vi "小灯泡控制pro.vi"() -> ()   [LabVIEW 2019]
panel:
  out "数值":i32
  out "布尔 2":bool
  in  "布尔":bool
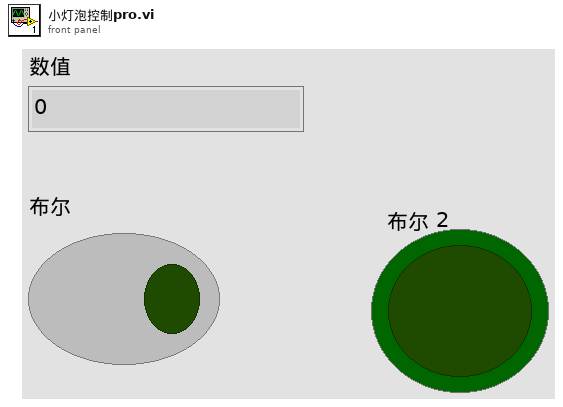
[diagram p1: front panel]
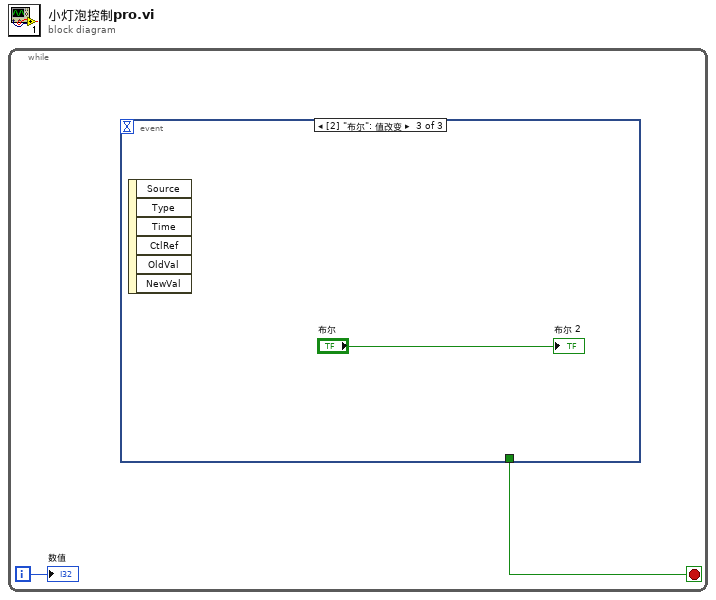
[diagram p0: block diagram]
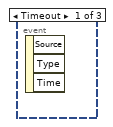
[diagram p2: hidden frame]
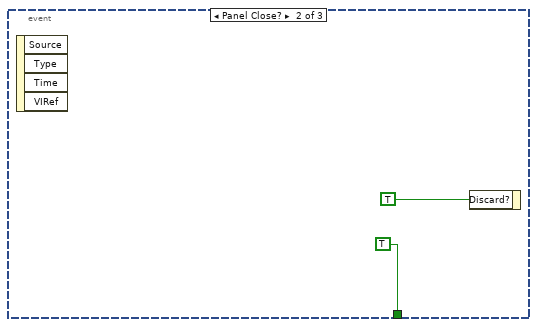
[diagram p3: hidden frame]
diagram:
  n1 = while {
    i -> [w2]
    stop <- w1 stop-if-true
    n2 = event shown="[2] \"布尔\": 值改变" {
      selector: _ -> [_ _ _]
      dyn-events: _ -> [_ _ _]
      timeout: _ -> [_ _ _]
      tunnel: [_ TRUE _] -> w1
      event Timeout {
        n3 = event-data() -> ()  [unwired: 1 in, 3 out]
      }
      event Panel Close? {
        n4 = event-data() -> ()  [unwired: 1 in, 4 out]
        n5 = event-data("Discard?"=TRUE ("放弃？")) -> ()  [unwired: 1 in, 1 out]
      }
      event "布尔": Value Change {
        n6 = event-data() -> ()  [unwired: 1 in, 6 out]
        "布尔 2" <- "布尔"
      }
    }
    "数值" <- w2
  }
